vi "Fit Transform.vi"(7 "Type X":T1(ring), 8 "error in (no error)":errorcluster caption="entrée d'erreur (pas d'erreur)", 9 "y":string[][](array[string]), 10 "X":string[][](array[string]), 11 "PolynomialFeatures.lvclass":refnum<class "PolynomialFeatures.lvclass">) -> (0 "error out":errorcluster caption="sortie d'erreur", 2 "Data":T2, 3 "PolynomialFeatures.lvclass":refnum<class "PolynomialFeatures.lvclass">)   [LabVIEW 2020, in "PolynomialFeatures.lvclass"]
doc: "Fit to data, then transform it.\n\nFits transformer to X and y with optional parameters fit_params and returns a transformed version of X.\n\nReturns : \n\n- X_new : ndarray array of shape (n_samples, n_features_new)\nTransformed array."
uses:
  PolynomialFeatures.lvclass
  PolynomialFeatures.lvclass/PolynomialFeatures.ctl
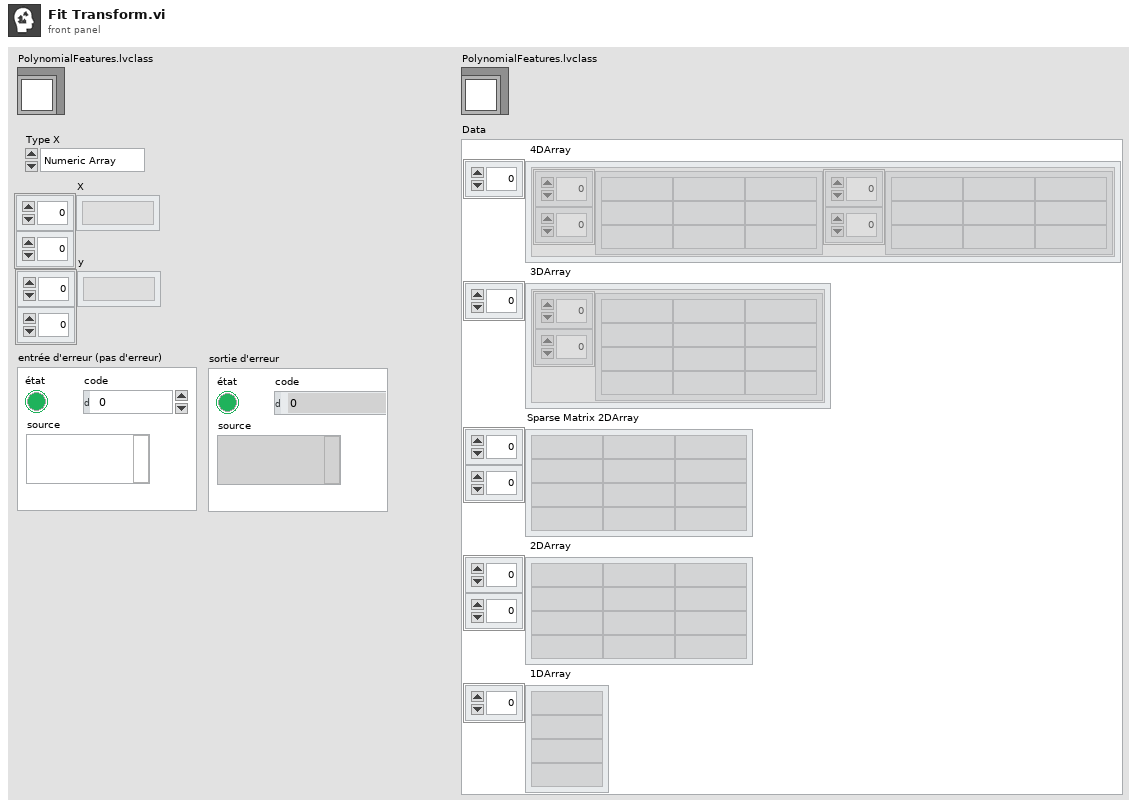
[diagram p1: front panel]
types:
  T1 = enum16{"Numeric Array", "String Array", "Sparse"}
  T2 = cluster{" 4DArray":cluster{"1":string[][], "2":string[][]}[], " 3DArray":cluster{"Tableau":string[][]}[], "Sparse Matrix 2DArray":string[][], " 2DArray":string[][], " 1DArray":string[]}
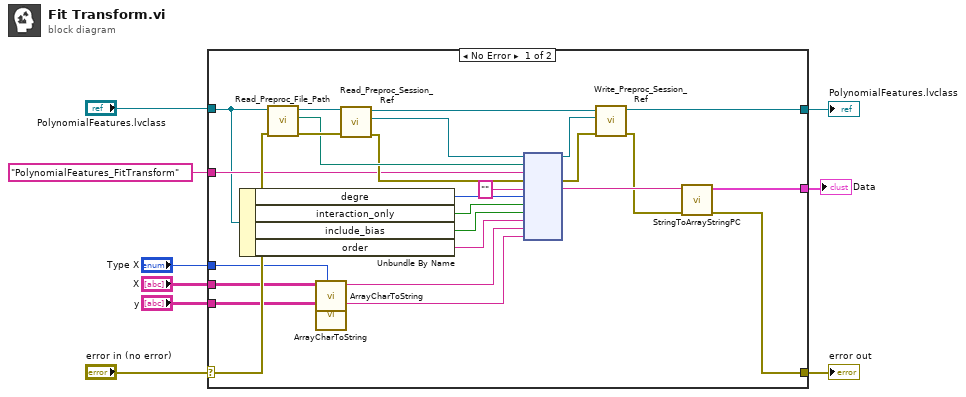
[diagram p0: block diagram]
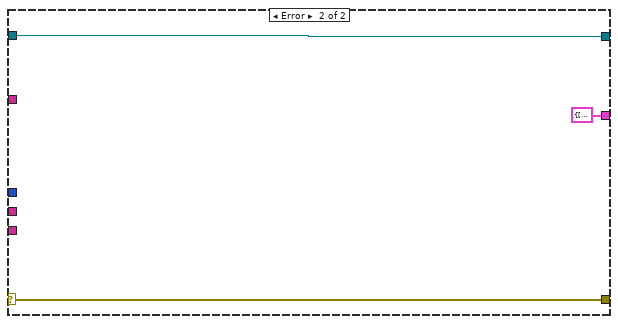
[diagram p2: hidden frame]
diagram:
  n1 = case shown="No Error" "error in (no error)" {
    selector: "error in (no error)" -> [w23 w38]
    tunnel: [w12 w38] -> w8
    tunnel: [w10 w37] -> w6
    tunnel: "PolynomialFeatures.lvclass" -> [w21 w37]
    tunnel: "PolynomialFeatures_FitTransform" ("Fonction") -> [w22 _]
    tunnel: [w11 T2 {" 4DArray"=[], " 3DArray"=[], "Sparse Matrix 2DArray"=[], " 2DArray"=[], " 1DArray"=[]} ("Data")] -> w4
    tunnel: "X" -> [w19 _]
    tunnel: "y" -> [w18 _]
    tunnel: "Type X" -> [w17 _]
    frame No Error {
      n2 = Unbundle By Name(w21) -> ("degre"=w26:i32, "interaction_only"=w25:bool, "include_bias"=w24:bool, "order"=w20:string)
      n3 = call-dynamic "Read_Preproc_File_Path.vi"("error in (no error)"=w23, "Python in"=w21) -> ("error out"=w34:errorcluster, "File_Path"=w31:path, "Python out"=w35:refnum<class "PolynomialFeatures.lvclass">)  [unwired: 7 in]
      n4 = call "ArrayCharToString.vi"("Type"=w17, "TAB"=w19) -> ("Instruction"=w16:string)  [unwired: 9 in]
      n5 = call "ArrayCharToString.vi"("TAB"=w18) -> ("Instruction"=w15:string)  [unwired: 10 in]
      n6 = call-dynamic "Read_Preproc_Session_Ref.vi"("error in (no error)"=w34, "Python in"=w35) -> ("error out"=w30:errorcluster, "Session_ref"=w32:refnum<k35>, "Python out"=w33:refnum<class "PolynomialFeatures.lvclass">)  [unwired: 7 in]
      n7 = node(w32, w31, w22, w30, "", w26, w25, w24, w20, w16, w15) -> (w28:refnum<k35>, w29:errorcluster, w14:string)  [unwired: 6 in, 2 out]
      n8 = call-dynamic "Write_Preproc_Session_Ref.vi"("error in (no error)"=w29, "Session_ref"=w28, "Python in"=w33) -> ("error out"=w13:errorcluster, "Python out"=w10:refnum<class "PolynomialFeatures.lvclass">)  [unwired: 7 in]
      n9 = call "StringToArrayStringPC.vi"("sortie d'erreur"=w13, "Return value"=w14) -> ("sortie d'erreur"=w12:errorcluster, "Data"=w11:T2)  [unwired: 8 in]
    }
    frame Error {
    }
  }
  "error out" <- w8
  "PolynomialFeatures.lvclass" <- w6
  "Data" <- w4
